vi "ActualizarCostosDB.vi"(8 "error in (no error)":errorcluster, 10 "COSTO":dbl, 11 "PRODUCTO":string) -> (0 "error out":errorcluster)   [LabVIEW 2020, in "DataBaseSQLlite.lvlib"]
uses:
  DataBaseSQLlite.lvlib
  <vilib>/drjdpowell/SQLite Library/SQL Connection/Open (path).vi
  <vilib>/drjdpowell/SQLite Library/SQL Connection/Open (string).vi
  <vilib>/AdvancedString/Path To Command Line String.vi
  <vilib>/drjdpowell/SQLite Library/SQL Connection/Execute SQL (No results).vi
  <vilib>/drjdpowell/SQLite Library/SQL Connection/Connection.lvclass
  <vilib>/drjdpowell/SQLite Library/SQLite.lvlib
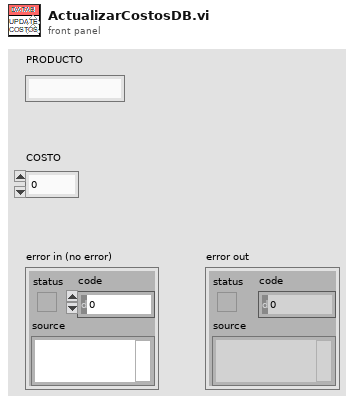
[diagram p1: front panel]
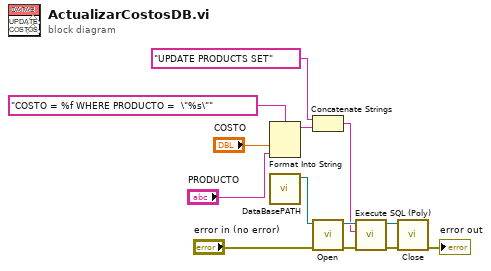
[diagram p0: block diagram]
diagram:
  n1 = Format Into String(format string="COSTO = %f WHERE PRODUCTO =  \"%s\"", "COSTO", "PRODUCTO") -> (resulting string=w10:string)  [unwired: 2 in, 1 out]
  n2 = call "DataBasePATH.vi"() -> ("DataBase path"=w8:path)  [unwired: 11 in]
  n3 = Concatenate Strings("UPDATE PRODUCTS SET" ("string"), w10) -> (w1:string)
  n4 = call-poly <vilib>:"Open.vi"("error in (no error)"="error in (no error)", "db file"=w8) -> ("error out"=w5:errorcluster, "SQLite Connection"=w6:refnum<class "Connection.lvclass">)  [unwired: 8 in]
  n5 = call-poly <vilib>:"Execute SQL (Poly).vi"("error in (no error)"=w5, "SQL"=w1, "SQLite Connection in"=w6) -> ("error out"=w3:errorcluster, "SQLite Connection"=w4:refnum<class "Connection.lvclass">)  [unwired: 7 in]
  n6 = call-dynamic "Close.vi"("error in (no error)"=w3, "SQLite Connection in"=w4) -> ("error out"=→"error out":errorcluster)  [unwired: 9 in]
